vi "temp.vi"(5 "Temp2 (Bottom) Port":tag="Dev2", 6 "Temp1 (Top) Port":tag="Dev1") -> (0 "error out":errorcluster caption="error out 1", 1 "Delta T":dbl, 2 "Bottom":dbl, 3 "Top":dbl, 4 "error out 2":errorcluster)   [LabVIEW 2015]
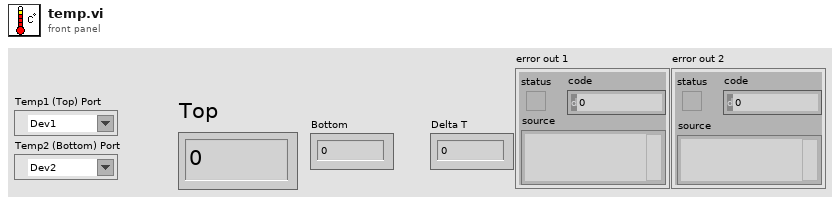
[diagram p1: front panel]
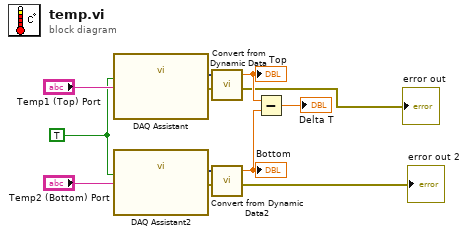
[diagram p0: block diagram]
diagram:
  w3 = TRUE ("stop (T)")
  n1 = call "DAQ Assistant"("stop (T)"=w3, "device name"="Temp1 (Top) Port") -> ("data"=w9:dynamicdata, "error out"=→"error out":errorcluster)  [unwired: 15 in, 1 out]
  n2 = call "DAQ Assistant2"("stop (T)"=w3, "device name"="Temp2 (Bottom) Port") -> ("data"=w10:dynamicdata, "error out"=→"error out 2":errorcluster)  [unwired: 15 in, 1 out]
  n3 = call "Convert from Dynamic Data"("Dynamic Data Type"=w9) -> ("Scalar"=w8:dbl)  [unwired: 3 in]
  "Top" <- w8
  n4 = call "Convert from Dynamic Data2"("Dynamic Data Type"=w10) -> ("Scalar"=w7:dbl)  [unwired: 3 in]
  "Bottom" <- w7
  n5 = Subtract(x=w8, y=w7) -> (x-y=→"Delta T":dbl)
